vi "Write maximum time (5s).vi"(8 "error in (no error)":errorcluster, 10 "maximum time (5s)":dbl[unit]=5000.0 caption="maximum time (5000 ms)", 11 "Read Multi-Point [MP] Msg in":refnum<class "Read Multi-Point [MP] Msg.lvclass">) -> (0 "error out":errorcluster, 3 "Read Multi-Point [MP] Msg out":refnum<class "Read Multi-Point [MP] Msg.lvclass">)   [LabVIEW 2015, in "CS++DMM.lvlib" / "Read Multi-Point [MP] Msg.lvclass"]
uses:
  Read Multi-Point [MP] Msg.lvclass
  Read Multi-Point [MP] Msg.lvclass/Read Multi-Point [MP] Msg.ctl
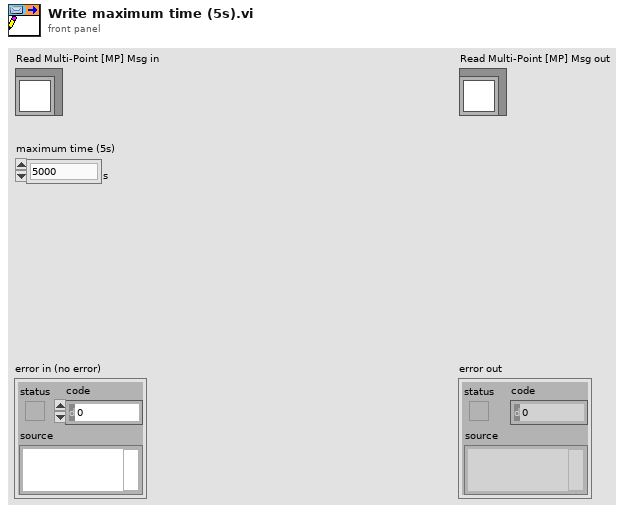
[diagram p1: front panel]
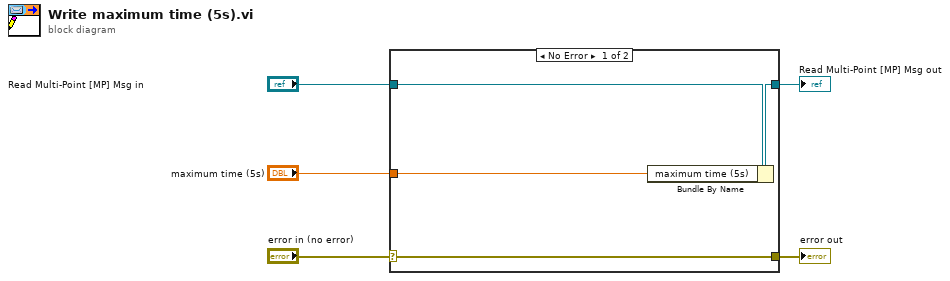
[diagram p0: block diagram]
diagram:
  n1 = case shown="No Error" "error in (no error)" {
    selector: "error in (no error)" -> [w9 w10]
    tunnel: [w9 w10] -> w4
    tunnel: [w7 w11] -> w2
    tunnel: "Read Multi-Point [MP] Msg in" -> [w8 w11]
    tunnel: "maximum time (5s)" -> [w6 _]
    frame No Error {
      n2 = Bundle By Name(cluster=w8, "maximum time (5s)"=w6) -> (w7:refnum<class "Read Multi-Point [MP] Msg.lvclass">)
    }
    frame Error {
    }
  }
  "error out" <- w4
  "Read Multi-Point [MP] Msg out" <- w2
